vi "Convert_Gauss_To_Tesla.vi"(10 "Name":string, 11 "historical trace in":cluster{"timestamps":timestamp[], "data":dbl[]}) -> (3 "historical trace out":cluster{"timestamps":timestamp[], "data":dbl[]})   [LabVIEW 2013]
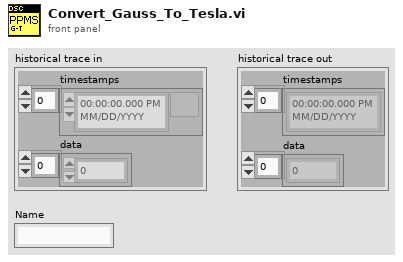
[diagram p1: front panel]
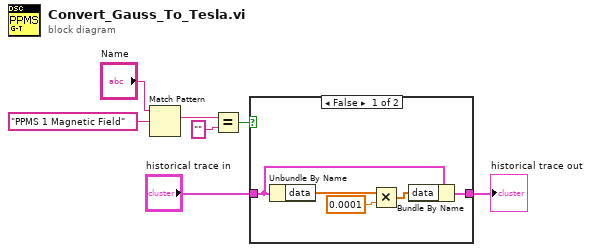
[diagram p0: block diagram]
diagram:
  n1 = Match Pattern(string="Name", regular expression="PPMS 1 Magnetic Field") -> (match substring=w2:string)  [unwired: 1 in, 3 out]
  n2 = Equal?(x=w2, y="") -> (x = y?=w4:bool)
  n3 = case shown="False" w4 {
    tunnel: "historical trace in" -> [w9 w13]
    tunnel: [w8 w13] -> w6
    frame False {
      n4 = Unbundle By Name(w9) -> ("data"=w11:dbl[])
      n5 = Multiply(x=w11, y=0.0001) -> (x*y=w10:dbl[])
      n6 = Bundle By Name(cluster=w9, "data"=w10) -> (w8:cluster{"timestamps":timestamp[], "data":dbl[]})
    }
    frame True {
    }
  }
  "historical trace out" <- w6
